vi "Pickup Floor.vi"(11 "Final Height":dbl format="%#_13g") -> ()   [LabVIEW 2014]
uses:
  Begin/Global Variables.vi
panel:
  in  "Slow":dbl=0.6
  in  "Fast":dbl=0.75
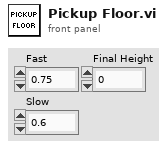
[diagram p1: front panel]
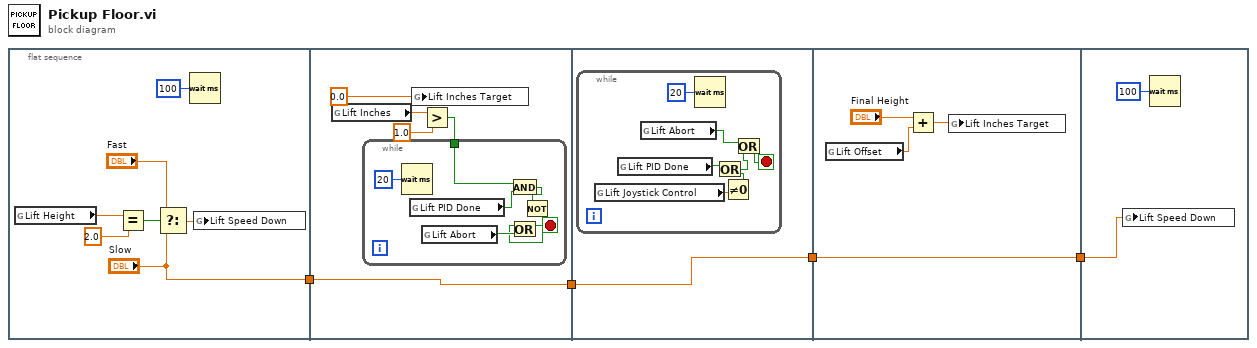
[diagram p0: block diagram]
diagram:
  n1 = flat-sequence {
    tunnel: ["Slow"] -> w1
    tunnel: [w12] -> w2
    tunnel: w1 -> [w12]
    tunnel: [w24] -> w3
    tunnel: w2 -> [w24]
    tunnel: [w32] -> w4
    tunnel: w3 -> [w32]
    tunnel: w4 -> [w36]
    frame #0 {
      n2 = global read "Global Variables.vi" "Lift Height"() -> (w10:dbl)
      n3 = Equal?(x=w10, y=2.0) -> (x = y?=w8:bool)
      n4 = Select(t="Fast", s=w8, f="Slow") -> (s? t:f=w7:dbl)
      n5 = Wait (ms)(milliseconds to wait=u32 100) -> ()  [unwired: 1 out]
      n6 = global write "Global Variables.vi" "Lift Speed Down"(w7) -> ()
    }
    frame #1 {
      n7 = global read "Global Variables.vi" "Lift Inches"() -> (w14:dbl)
      n8 = global write "Global Variables.vi" "Lift Inches Target"(0.0 ("x")) -> ()
      n9 = Greater?(x=w14, y=1.0) -> (0:w13:bool)
      n10 = while {
        tunnel: w13 -> [w21]
        stop <- w19 stop-if-true
        n11 = Wait (ms)(milliseconds to wait=u32 20) -> ()  [unwired: 1 out]
        n12 = global read "Global Variables.vi" "Lift PID Done"() -> (w22:bool)
        n13 = global read "Global Variables.vi" "Lift Abort"() -> (w18:bool)
        n14 = And(x=w21, y=w22) -> (x .and. y?=w20:bool)
        n15 = Not(x=w20) -> (.not. x?=w17:bool)
        n16 = Or(x=w17, y=w18) -> (x .or. y?=w19:bool)
      }
    }
    frame #2 {
      n17 = while {
        stop <- w26 stop-if-true
        n18 = global read "Global Variables.vi" "Lift Joystick Control"() -> (w30:dbl)
        n19 = global read "Global Variables.vi" "Lift PID Done"() -> (w28:bool)
        n20 = global read "Global Variables.vi" "Lift Abort"() -> (w25:bool)
        n21 = Wait (ms)(milliseconds to wait=u32 20) -> ()  [unwired: 1 out]
        n22 = Not Equal To 0?(x=w30) -> (x != 0?=w29:bool)
        n23 = Or(x=w28, y=w29) -> (x .or. y?=w27:bool)
        n24 = Or(x=w25, y=w27) -> (x .or. y?=w26:bool)
      }
    }
    frame #3 {
      n25 = global read "Global Variables.vi" "Lift Offset"() -> (w34:dbl)
      n26 = Add(x="Final Height", y=w34) -> (x+y=w35:dbl)
      n27 = global write "Global Variables.vi" "Lift Inches Target"(w35) -> ()
    }
    frame #4 {
      n28 = global write "Global Variables.vi" "Lift Speed Down"(w36) -> ()
      n29 = Wait (ms)(milliseconds to wait=u32 100) -> ()  [unwired: 1 out]
    }
  }
